vi "Offset_decoder_with_sign_CH0.vi"(11 "Array In1":dbl[](array[numeric])) -> (2 "Sign":dbl format="%.2f", 3 "CH0 uV":dbl)   [LabVIEW 2012]
panel:
  out "6 sign":dbl format="%.2f"
  out "4":dbl format="%.2f"
  out "5":dbl format="%.2f"
  # "Byte 2,3,4,5: Shift voltage CH0"
  # "CH0 LB"
  # "2"
  # "CH0 HB"
  # "CH0 UB"
  # "CH0 MB"
  # "CH0 sign"
  # "CH1 LB"
  # "CH1 HB"
  # "CH1 UB"
  # "CH1 MB"
  # "CH1 sign"
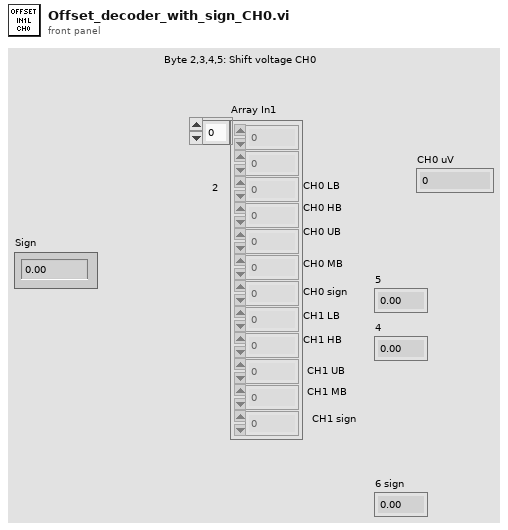
[diagram p1: front panel]
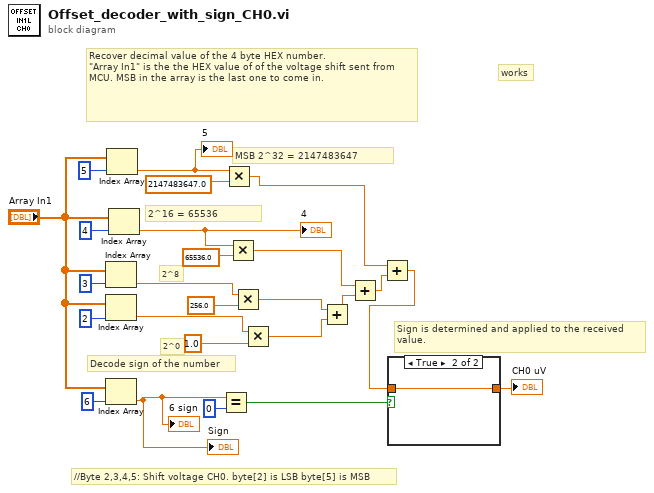
[diagram p0: block diagram]
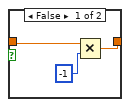
[diagram p2: hidden frame]
diagram:
  # "works"
  # "//Byte 2,3,4,5: Shift voltage CH0. byte[2] is LSB byte[5] is MSB"
  # "Decode sign of the number"
  # "Recover decimal value of the 4 byte HEX number.\n\"Array In1\" is the the HEX value of of the voltage shift sent from MCU. MSB in the array is the last one to come in."
  # "Sign is determined and applied to the received \nvalue."
  # "2^0"
  # "2^8"
  # "2^16 = 65536"
  # "MSB 2^32 = 2147483647"
  n1 = Index Array(array="Array In1", index=3) -> (element=w1:dbl)
  n2 = Index Array(array="Array In1", index=2) -> (element=w3:dbl)
  n3 = Index Array(array="Array In1", index=6) -> (element=w2:dbl)
  "Sign" <- w2
  "6 sign" <- w2
  n4 = Index Array(array="Array In1", index=5) -> (element=w5:dbl)
  "5" <- w5
  n5 = Index Array(array="Array In1", index=4) -> (element=w4:dbl)
  "4" <- w4
  n6 = Equal?(x=w2, y=u8 0) -> (x = y?=w15:bool)
  n7 = Multiply(x=w5, y=2147483647.0) -> (x*y=w12:dbl)
  n8 = Multiply(x=w4, y=65536.0) -> (x*y=w19:dbl)
  n9 = Multiply(x=w1, y=256.0) -> (x*y=w22:dbl)
  n10 = Multiply(x=w3, y=1.0) -> (x*y=w21:dbl)
  n11 = Add(x=w22, y=w21) -> (x+y=w20:dbl)
  n12 = Add(x=w19, y=w20) -> (x+y=w18:dbl)
  n13 = Add(x=w12, y=w18) -> (x+y=w13:dbl)
  n14 = case shown="True" w15 {
    tunnel: w13 -> [w26 w29]
    tunnel: [w28 w29] -> w10
    frame False {
      n15 = Multiply(x=w26, y=-1) -> (x*y=w28:dbl)
    }
    frame True {
    }
  }
  "CH0 uV" <- w10
